vi "refreshLabviewMenus.vi"   [LabVIEW 2017, in "ide_tools.lvlib"]
doc: "Refreshes the File, Tools, and Help menus from disk."
uses:
  ide_tools.lvlib
panel:
  # "Pleasewait while we refresh the LabVIEW File, Tools, and Help menus."
types:
  T1 = enum32{"Invalid", "Standard", "Closed", "Hidden", "Minimized", "Maximized"}
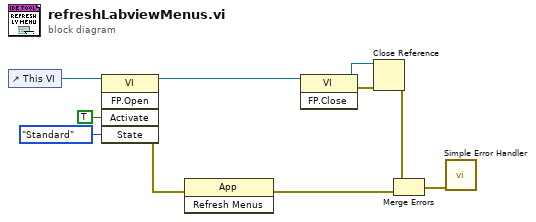
[diagram p0: block diagram]
diagram:
  n1 = control-ref of="This VI"() -> (w10:refnum<vi>)
  n2 = invoke on="Invoke Node" class="VI" method="FP.Open"(reference=w10, "Activate"=TRUE ("Activate?"), "State"=T1."Standard") -> (reference out=w6:refnum<vi>, error out=w7:errorcluster)  [unwired: 2 in, 3 out]
  n3 = invoke on="Invoke Node" class="App" method="Refresh Menus"(error in=w7) -> (error out=w4:errorcluster)  [unwired: 2 in, 2 out]
  n4 = invoke on="Invoke Node" class="VI" method="FP.Close"(reference=w6) -> (reference out=w1:refnum<vi>, error out=w3:errorcluster)  [unwired: 2 in, 1 out]
  n5 = Close Reference(reference=w1, error in (no error)=w3) -> (error out=w2:errorcluster)
  n6 = Merge Errors(w2, w4) -> (w5:errorcluster)
  n7 = call <vilib>:"Simple Error Handler.vi"("error in (no error)"=w5) -> ()  [unwired: 4 in, 5 out]
